vi "Power Meter Read Power (No Objects).vi"(8 "error in (no error)":errorcluster, 11 "Cluster In":T2={"Wavelength"=0.0, "AVG"=0, "Range"=0, "Backlight"=0, "Beeper"=0, "Zero"=0, "Local Lockout"=0, "ATTN"=0, "Run/Stop"=0, "Units"=0, "Averaging Time"=0.5, "Averaging"=FALSE, "Most Recent Power"=5.5, "Filter"=1} {"AVG" items=["Slow"=1, "Medium"=2, "Fast"=3]; "Range" items=["Auto", "Lowest", "2", "3", "4", "5", "6", "7", "Highest"]; "Backlight" items=["Off", "Low", "High"]; "Beeper" items=["Off", "On"]; "Zero" items=["Off", "On"]; "Local Lockout" items=["Off", "On"]; "ATTN" items=["Off", "On"]; "Run/Stop" items=["Stop", "Run"]; "Units" items=["W"=1, "dB"=2, "dBm"=3, "REL"=4]; "Filter" items=["Orange"=1, "Green"=2, "Yellow"=3]}) -> (0 "error out":errorcluster, 1 "Current Power w/ Units":string, 2 "Current Power":dbl[unit], 3 "Cluster Out":T2={"Wavelength"=0.0, "AVG"=0, "Range"=0, "Backlight"=0, "Beeper"=0, "Zero"=0, "Local Lockout"=0, "ATTN"=0, "Run/Stop"=0, "Units"=0, "Averaging Time"=0.5, "Averaging"=FALSE, "Most Recent Power"=5.5, "Filter"=1} {"AVG" items=["Slow"=1, "Medium"=2, "Fast"=3]; "Range" items=["Auto", "Lowest", "2", "3", "4", "5", "6", "7", "Highest"]; "Backlight" items=["Off", "Low", "High"]; "Beeper" items=["Off", "On"]; "Zero" items=["Off", "On"]; "Local Lockout" items=["Off", "On"]; "ATTN" items=["Off", "On"]; "Run/Stop" items=["Stop", "Run"]; "Units" items=["W"=1, "dB"=2, "dBm"=3, "REL"=4]; "Filter" items=["Orange"=1, "Green"=2, "Yellow"=3]})   [LabVIEW 2009]
doc: "Advanced Read for Power Meter.\n\nPerforms time-based Averaging based of member data. Checks for erroneous data points due to auto-ranging. Also has formatted power output."
uses:
  Newport 1830-C/Public/Filters.ctl
  Global/GPIB Numbers.vi
  Newport 1830-C/Newport 1830-C.lvlib
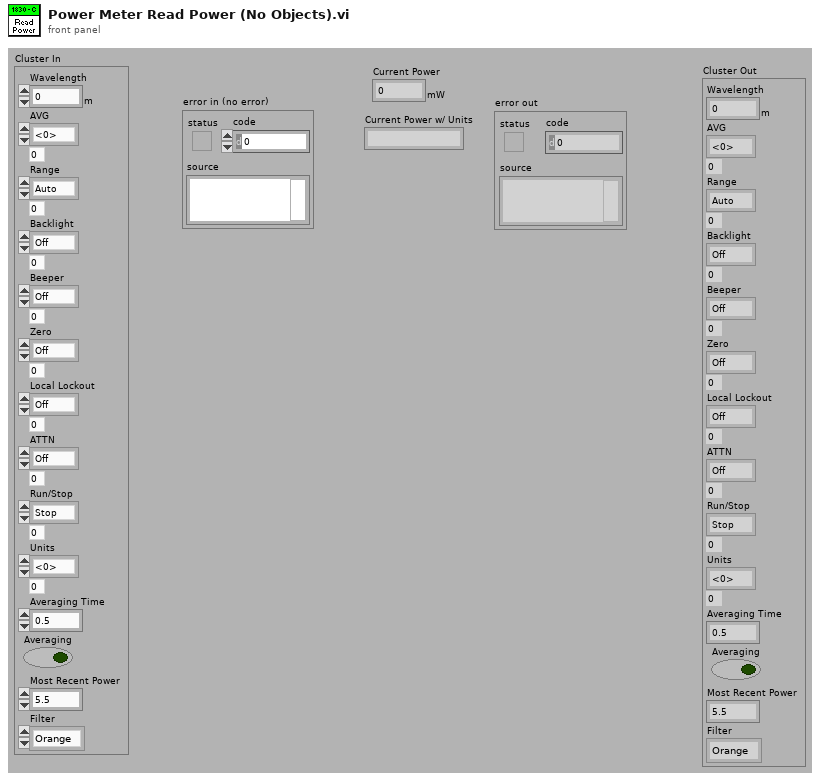
[diagram p1: front panel]
types:
  T1 = typedef "Filters.ctl" = u16
  T2 = cluster{"Wavelength":dbl[unit], "AVG":u16, "Range":u16, "Backlight":u16, "Beeper":u16, "Zero":u16, "Local Lockout":u16, "ATTN":u16, "Run/Stop":u16, "Units":u16, "Averaging Time":dbl, "Averaging":bool, "Most Recent Power":dbl, "Filter":T1}
  T3 = typedef "GPIB Type Def.ctl" = cluster{"Name":string, "bus":dbl, "GPIB":dbl, "GPIB as string":string, "byte":i32, "VISA Resource Name":refnum<visa-resource-name>}
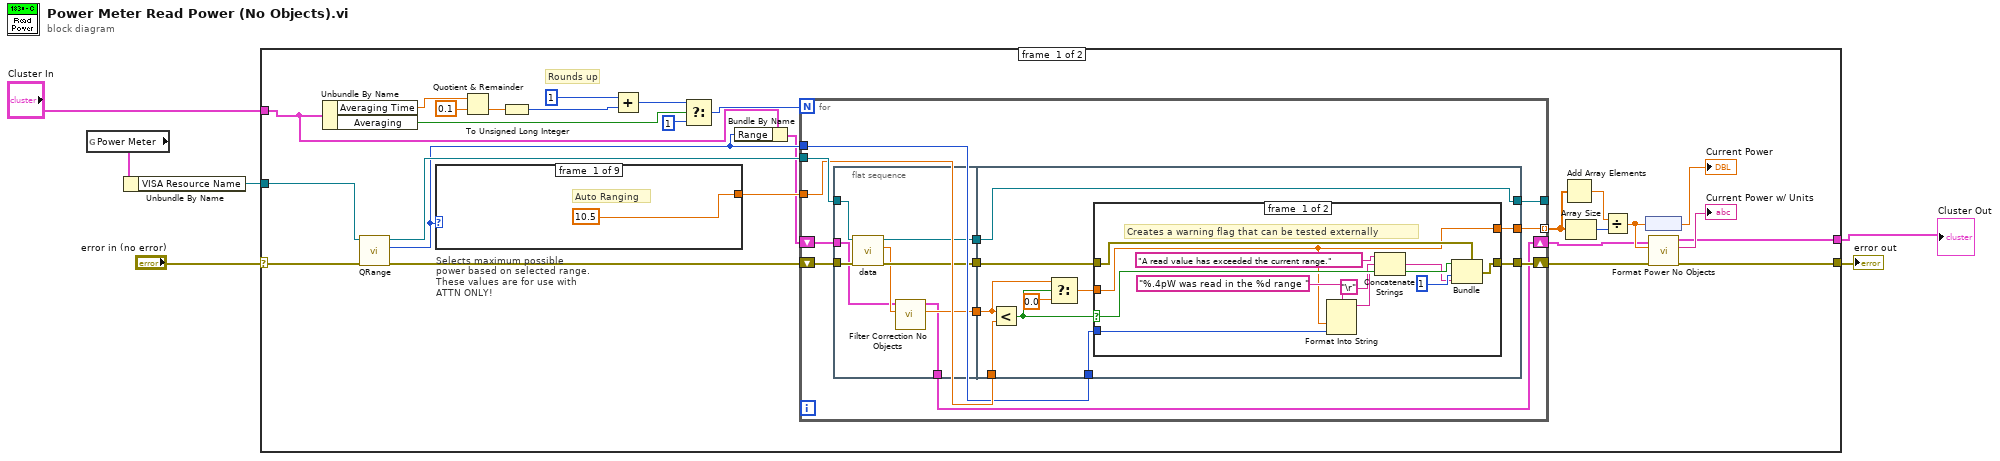
[diagram p0: block diagram]
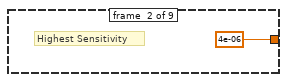
[diagram p2: hidden frame]
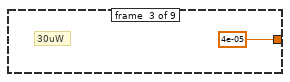
[diagram p3: hidden frame]
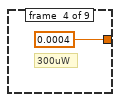
[diagram p4: hidden frame]
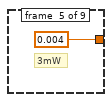
[diagram p5: hidden frame]
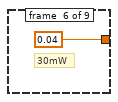
[diagram p6: hidden frame]
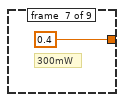
[diagram p7: hidden frame]
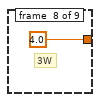
[diagram p8: hidden frame]
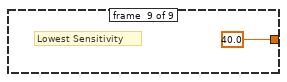
[diagram p9: hidden frame]
diagram:
  n1 = global read "GPIB Numbers.vi" "Power Meter"() -> (w4:T3)
  n2 = Unbundle By Name(w4) -> ("VISA Resource Name"=w3:refnum<visa-resource-name>)
  n3 = case shown="No Error" "error in (no error)" {
    selector: "error in (no error)" -> [w10 w87]
    tunnel: [w7 w87] -> w5
    tunnel: [w8 w86] -> w1
    tunnel: w3 -> [w12 _]
    tunnel: "Cluster In" -> [w11 w86]
    frame #0 {
      # "Rounds up"
      n4 = Unbundle By Name(w11) -> ("Averaging Time"=w22:dbl, "Averaging"=w23:bool)
      n5 = call "QRange.vi"("error in (no error)"=w10, "VISA resource name"=w12) -> ("error out"=w17:errorcluster, "Range"=w14:u32, "VISA resource name out"=w18:refnum<visa-resource-name>)  [unwired: 7 in]
      n6 = case "Selects maximum possible\npower based on selected range.\nThese values are for use with\nATTN ONLY!" shown="4" w14 {
        tunnel: [10.5 ("y") 4e-06 ("y") 4e-05 ("y") 0.0004 ("y") 0.004 ("y") 0.04 ("y") 0.4 ("y") 4.0 ("y") 40.0 ("y")] -> w16
        frame #0 {
          # "Auto Ranging"
        }
        frame #1 {
          # "Highest Sensitivity"
        }
        frame #2 {
          # "30uW"
        }
        frame #3 {
          # "300uW"
        }
        frame #4 {
          # "3mW"
        }
        frame #5 {
          # "30mW"
        }
        frame #6 {
          # "300mW"
        }
        frame #7 {
          # "3W"
        }
        frame #8 {
          # "Lowest Sensitivity"
        }
      }
      n7 = Quotient & Remainder(x=w22, y=0.1) -> (floor(x/y)=w27:dbl)  [unwired: 1 out]
      n8 = To Unsigned Long Integer(number=w27) -> (unsigned 32bit integer=w26:u32)
      n9 = Add(x=u32 1, y=w26) -> (x+y=w30:u32)
      n10 = Select(t=w30, s=w23, f=u32 1 ("t")) -> (s? t:f=w24:u32)
      n11 = Bundle By Name(cluster=w11, "Range"=w14) -> (w13:T2)
      n12 = for {
        N: w24 -> [_]
        tunnel: w18 -> [w54]
        tunnel: [w52] -> _
        tunnel: w16 -> [w47]
        tunnel: w14 -> [w46]
        tunnel: [w45] -> w15 mode=indexing
        shift-right: [w51] -> w21
        shift-left: w17 -> [w53]
        shift-right: [w43] -> w9
        shift-left: w13 -> [w44]
        n13 = flat-sequence {
          tunnel: w54 -> [w62]
          tunnel: w53 -> [w61]
          tunnel: [w60] -> w50
          tunnel: [w59] -> w49
          tunnel: [w57] -> w48
          tunnel: w44 -> [w55]
          tunnel: [w56] -> w43
          tunnel: [w69] -> w51
          tunnel: [w72] -> w52
          tunnel: w50 -> [w72]
          tunnel: w49 -> [w70]
          tunnel: w48 -> [w67]
          tunnel: w47 -> [w68]
          tunnel: w46 -> [w65]
          tunnel: [w64] -> w45
          frame #0 {
            n14 = call "data.vi"("error in (no error)"=w61, "VISA resource name"=w62) -> ("error out"=w59:errorcluster, "Power"=w58:dbl, "VISA resource name out"=w60:refnum<visa-resource-name>)  [unwired: 7 in]
            n15 = call "Filter Correction No Objects.vi"("Read Power"=w58, "Cluster In"=w55) -> ("Corrected Power"=w57:dbl, "Cluster Out"=w56:T2)  [unwired: 8 in]
          }
          frame #1 {
            n16 = Less?(x=w67, y=w68) -> (x < y?=w63:bool)
            n17 = Select(t=w67, s=w63, f=0.0) -> (s? t:f=w66:dbl)
            n18 = case shown="False" w63 {
              selector: w63 -> [w82 _]
              tunnel: w70 -> [w83 w85]
              tunnel: [w80 w85] -> w69
              tunnel: w66 -> [w75 w84]
              tunnel: w65 -> [w76 _]
              tunnel: [w75 w84] -> w64
              frame #0 {
                # "Creates a warning flag that can be tested externally"
                n19 = Format Into String(format string="%.4pW was read in the %d range ", w75, w76) -> (resulting string=w74:string)  [unwired: 2 in, 1 out]
                n20 = Concatenate Strings("A read value has exceeded the current range." ("source"), "\r", w74) -> (w77:string)
                n21 = Bundle(cluster=w83, "status"=w82, "code"=1, "source"=w77) -> (w80:errorcluster)
              }
              frame #1 {
              }
            }
          }
        }
      }
      n22 = Add Array Elements(numeric array=w15) -> (sum=w31:dbl)
      n23 = Array Size(array=w15) -> (size(s)=w32:i32)
      n24 = Divide(x=w31, y=w32) -> (x/y=w20:dbl)
      n25 = node(w20) -> (→"Current Power":dbl[unit])
      n26 = call "Format Power No Objects.vi"("error in"=w21, "Power"=w20, "Cluster In"=w9) -> ("error out"=w7:errorcluster, "Formatted Power"=→"Current Power w/ Units":string, "Cluster Out"=w8:T2)  [unwired: 6 in]
    }
    frame #1 {
    }
  }
  "error out" <- w5
  "Cluster Out" <- w1
